vi "多参数全局变量.vi"() -> ()   [LabVIEW 2016, in "斯坦道多参数.lvlib"]
uses:
  <vilib>/Plasmionique/MB Master/MB_Master/MB_Master.lvclass
panel:
  out "禹山KB值":T1
  out "重新获取KB值命令":bool
  in  "校准参数":u16(ring) caption="校准参数：" items=["pH", "DO", "浊度", "电导率"]
  out "多参数水样测试值":T2
  in  "当前页面":enum16{"主页面", "参数页面", "校准页面"}(ring)
  in  "权限密码":u32[](array[numeric])=[0, 23506, 783523506, 783523103]
  out "DO2显示":T3
  out "DO2通讯状态":bool
  out "启动参数名称":string[](array[string])
  in  "数据标识":string
  out "cod通讯状态":bool
  out "COD显示":T4
  out "远程校准运行状态":T5
  out "校准运行状态":T6
  in  "权限":enum16{"一级权限", "二级权限", "三级权限", "超级权限"}(ring)
  out "ORP显示":T4
  out "orp通讯状态":bool
  out "蓝绿藻通讯状态":bool
  out "藻密度通讯状态":bool
  out "叶绿素a通讯状态":bool
  out "浊度通讯状态":bool
  out "spcond通讯状态":bool
  out "DO通讯状态":bool
  out "ph通讯状态":bool
  in  "MB session in":refnum<class "MB_Master.lvclass">
  in  "多参数编号":string
  out "藻密度显示":T4
  out "蓝绿藻显示":T4
  out "cond显示":T4
  out "盐度显示":T4
  out "spcond显示":T4
  out "ph显示":T4
  out "水温显示":T7={"CH"=1, "监测值"=0.0, "信号值"=0.0, "数据标识"=""} {"CH" items=["pH", "DO", "浊度", "叶绿素a", "藻密度"]}
  out "浊度显示":T4
  out "DO显示":T3
  out "叶绿素a显示":T4
  out "多参数运行状态":u16(ring) items=["空闲", "水样测试", "标样核查"]
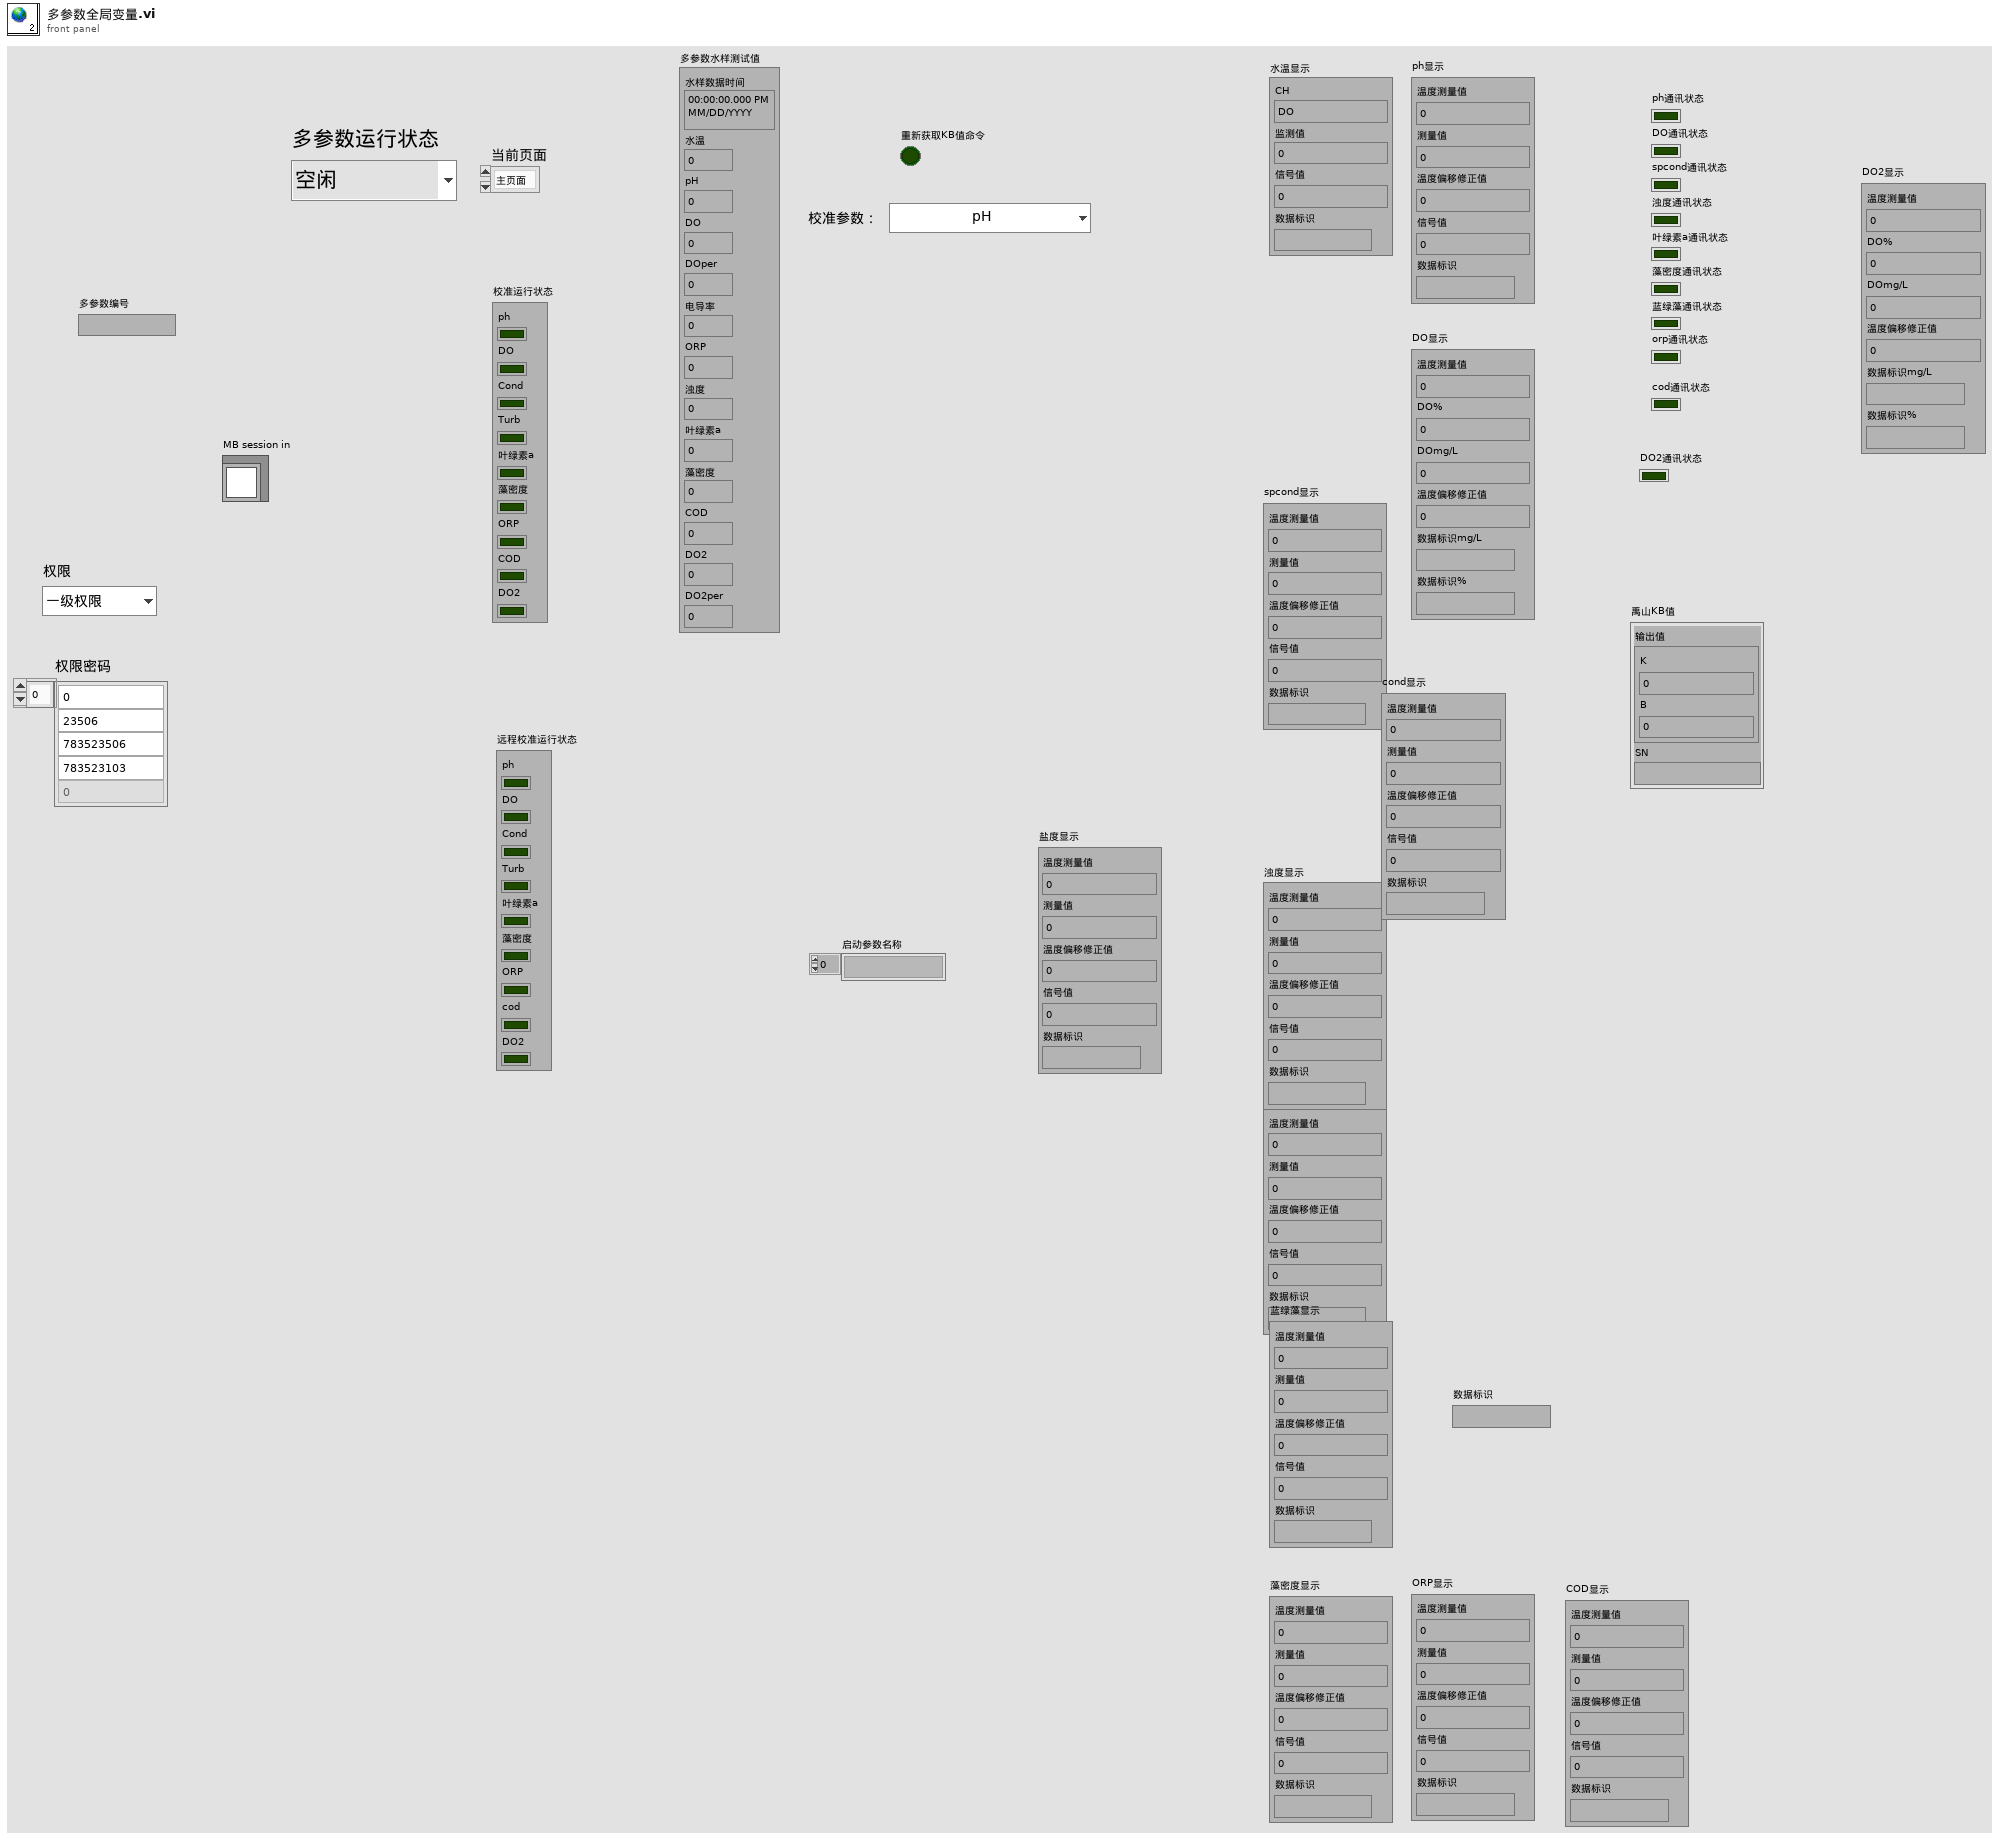
[diagram p1: front panel]
types:
  T1 = cluster{"输出值":cluster{"K":sgl, "B":sgl}, "SN":string}
  T2 = cluster{"水样数据时间":timestamp, "水温":dbl, "pH":dbl, "DO":dbl, "DOper":dbl, "电导率":dbl, "ORP":dbl, "浊度":dbl, "叶绿素a":dbl, "藻密度":dbl, "COD":dbl, "DO2":dbl, "DO2per":dbl}
  T3 = cluster{"温度测量值":sgl, "DO%":sgl, "DOmg/L":sgl, "温度偏移修正值":sgl, "数据标识mg/L":string, "数据标识%":string}
  T4 = cluster{"温度测量值":sgl, "测量值":sgl, "温度偏移修正值":sgl, "信号值":sgl, "数据标识":string}
  T5 = cluster{"ph":bool, "DO":bool, "Cond":bool, "Turb":bool, "叶绿素a":bool, "藻密度":bool, "ORP":bool, "cod":bool, "DO2":bool}
  T6 = cluster{"ph":bool, "DO":bool, "Cond":bool, "Turb":bool, "叶绿素a":bool, "藻密度":bool, "ORP":bool, "COD":bool, "DO2":bool}
  T7 = cluster{"CH":u16, "监测值":dbl, "信号值":sgl, "数据标识":string}
diagram:
